vi "property node.vi"() -> ()   [LabVIEW 2013]
uses:
  <vilib>/userDefined/High Color/IMAQdx.ctl
  <vilib>/vision/driver/NI_Vision_Acquisition_Software.lvlib
  <resource>/objmgr/imaqdx.rc
panel:
  out "Image":T1(plugin-control)
  in  "Gain":dbl
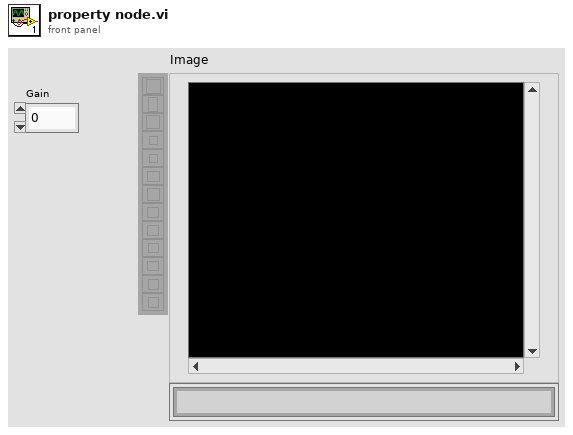
[diagram p1: front panel]
types:
  T1 = typedef "IMAQ Image.ctl" = refnum<image>
  T2 = typedef "IMAQdx.ctl" = refnum<k21>
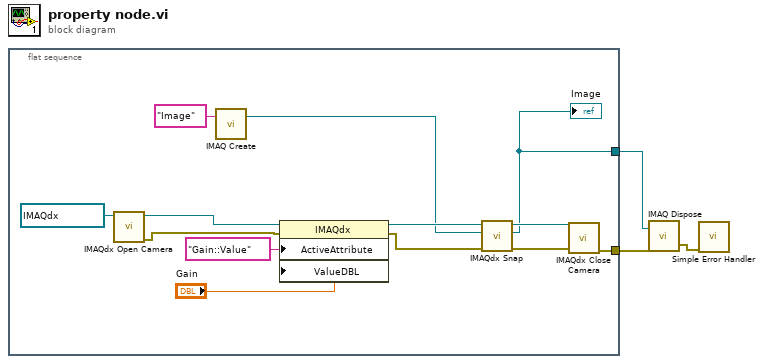
[diagram p0: block diagram]
diagram:
  n1 = flat-sequence {
    tunnel: [w5] -> w3
    tunnel: [w4] -> w1
    frame #0 {
      n2 = call <vilib>:"IMAQdx Open Camera.vi"("Session In"=T2 "cam0") -> ("error out"=w11:errorcluster, "Session Out"=w15:T2)  [unwired: 9 in]
      n3 = call "IMAQ Create"("Image Name"="Image") -> ("New Image"=w9:T1)  [unwired: 4 in, 1 out]
      n4 = property class="IMAQdx"(reference=w15, error in=w11, "ActiveAttribute"="Gain::Value", "ValueDBL"="Gain") -> (reference out=w10:T2, error out=w8:errorcluster)
      n5 = call <vilib>:"IMAQdx Snap.vi"("error in"=w8, "Image In"=w9, "Session In"=w10) -> ("error out"=w7:errorcluster, "Image Out"=w4:T1, "Session Out"=w6:T2)  [unwired: 6 in]
      "Image" <- w4
      n6 = call <vilib>:"IMAQdx Close Camera.vi"("error in"=w7, "Session In"=w6) -> ("error out"=w5:errorcluster)  [unwired: 9 in]
    }
  }
  n7 = call "IMAQ Dispose"("Image"=w1, "error in (no error)"=w3) -> ("error out"=w2:errorcluster)  [unwired: 4 in]
  n8 = call <vilib>:"Simple Error Handler.vi"("error in (no error)"=w2) -> ()  [unwired: 4 in, 5 out]
